vi "Debouncing.vi"(8 "error in":errorcluster, 11 "Input Signal":bool) -> (0 "error out":errorcluster, 3 "Filtered Signal":bool)   [LabVIEW 2014]
panel:
  in  "Cycles to Filter":i32=10
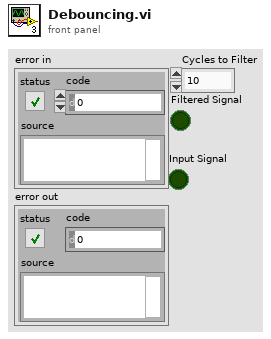
[diagram p1: front panel]
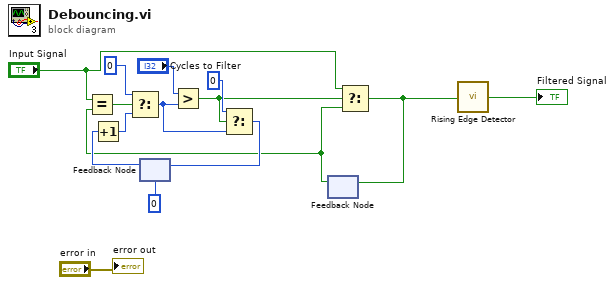
[diagram p0: block diagram]
diagram:
  n1 = feedback #1(0) -> (w8:i32)
  n2 = Increment(x=w8) -> (x+1=w7:i32)
  n3 = feedback #2() -> (w3:bool)  [unwired: 1 in]
  n4 = Equal?(x="Input Signal", y=w3) -> (x = y?=w14:bool)
  n5 = Select(t=0, s=w14, f=w7) -> (s? t:f=w10:i32)
  n6 = Greater?(x="Cycles to Filter", y=w10) -> (0:w5:bool)
  n7 = Select(t=0, s=w5, f=w10) -> (s? t:f=w9:i32)
  n8 = feedback-in #1(w9) -> ()
  n9 = Select(t="Input Signal", s=w5, f=w3) -> (s? t:f=w2:bool)
  n10 = feedback-in #2(w2) -> ()
  n11 = call "Rising Edge Detector.vi"("Input"=w2) -> ("Rising edge?"=→"Filtered Signal":bool)
  "error out" <- "error in"
